vi "OAT_Display_Freq-RPM Map.vi"(9 "Gabor Template":dbl[](array[numeric]) format="%.2f", 10 "sampling frequency (Hz)":dbl, 11 "Gabor RefNum":T1) -> (1 "Diagram":picture, 2 "Freq-RPM Map":u8[][](graph), 3 "Gabor RefNum Out":T1, 4 "Diagram":bool, 5 "Order":dbl=1.0 format="%.1f")   [LabVIEW 2017]
doc: "This VI is a sub-window of Order Analyzer. It displays RPM-Order map in intensity graph and waterfall plot."
uses:
  <vilib>/addons/Sound and Vibration/Order Analysis/Ref Gabor Order Tracking/GT RefNum.ctl
  <vilib>/addons/Sound and Vibration/Order Analysis/Ref Gabor Order Tracking/Get Freq-RPM Spectral Map (DBL).vi
  <vilib>/addons/Sound and Vibration/Order Analysis/Ref Gabor Order Tracking/Get Freq-RPM Spectral Map (U8).vi
  <vilib>/addons/Sound and Vibration/Order Analysis/Gabor Order Tracking/SoundVib_Gabor.lvlib
panel:
  in  "help mask":cluster{"OK Button":bool}
  in  "Help":bool
  out "Cursor Mask":cluster{dbl, dbl}[](graph)
  in  "stop":bool
  in  "[user-specified font]":T2={"Font Name:"="MS Sans Serif", "Size"=13, "Strikeout?"=FALSE, "Italic?"=FALSE, "Underline?"=FALSE, "Outline?"=FALSE, "Shadow?"=FALSE, "Bold?"=FALSE}
  in  "Order Info":T3={"Lowest order"=1.0, "# of Orders"=20.0, "Resolution"=0.1} {"Resolution" format="%.2f"; "# of Orders" format="%.1f"; "Lowest order" format="%.1f"}
  in  "dB ON":bool=TRUE
  in  "Waterfall ColorMap":i32(ring)=2 items=["cwNone", "cwShaded", "cwColorSpectrum", "cwGrayScale"]
  out "status":string
  in  "Diagram\n\nIntensity":bool
  # "1. Zoom Intensity Graph by setting ranges of axis.\n\n2. Switch to Diagram to display Campbell diagram.\n\n3. Move the cursor to find out which order the engergy consentrats on.\n\nClick on this screen to continue"
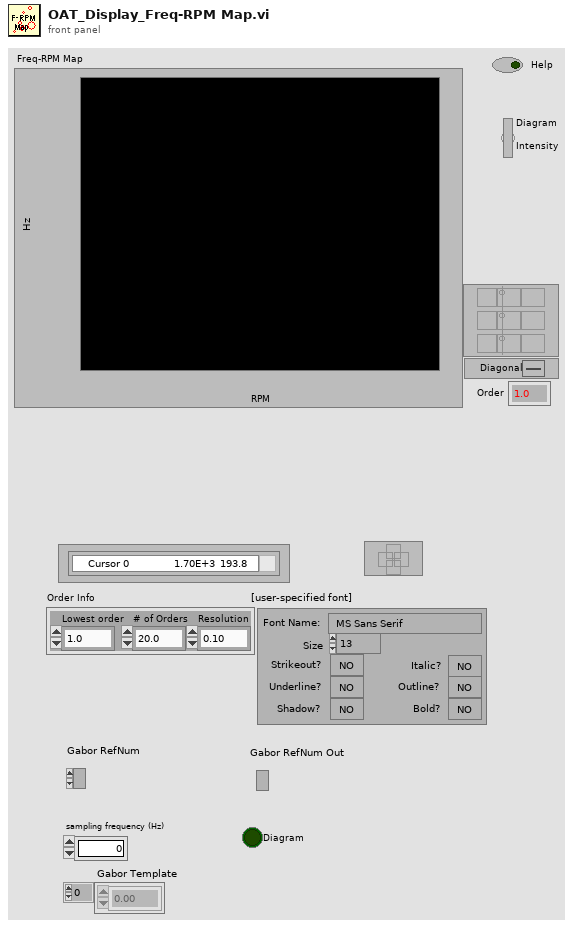
[diagram p1: front panel]
types:
  T1 = typedef "SoundVib_Gabor.lvlib/GT RefNum.ctl" = refnum<k1>
  T2 = cluster{"Font Name:":string, "Size":i16, "Strikeout?":bool, "Italic?":bool, "Underline?":bool, "Outline?":bool, "Shadow?":bool, "Bold?":bool}
  T3 = cluster{"Lowest order":dbl, "# of Orders":dbl, "Resolution":dbl}
  T4 = enum16{"User-specified Font", "Application Font", "System Font", "Dialog Font"}
  T5 = cluster{"x minimum":dbl, "x maximum":dbl, "x log?":bool, "x precision":u8, "x format":enum8{"Decimal", "Scientific", "Engineering", "Binary", "Octal", "Hex"}, "y minimum":dbl, "y maximum":dbl, "y log?":bool, "y precision":u8, "y format":enum8{"Decimal", "Scientific", "Engineering", "Binary", "Octal", "Hex"}}
  T6 = cluster{"Gabor RefNum":T1, "dB ON":bool, "Order Info":cluster{"Lowest order":dbl, "# of Orders":dbl, "Resolution":dbl}}
  T7 = cluster{"Diagram\n\nIntensity":bool, "Waterfall ColorMap":i32}
  T8 = typedef "LVBoundsTypeDef.ctl" = cluster{"Width":u32, "Height":u32}
  T9 = cluster{"x [EU]":dbl, "y [EU]":dbl, "radius [pixel]":dbl}[]
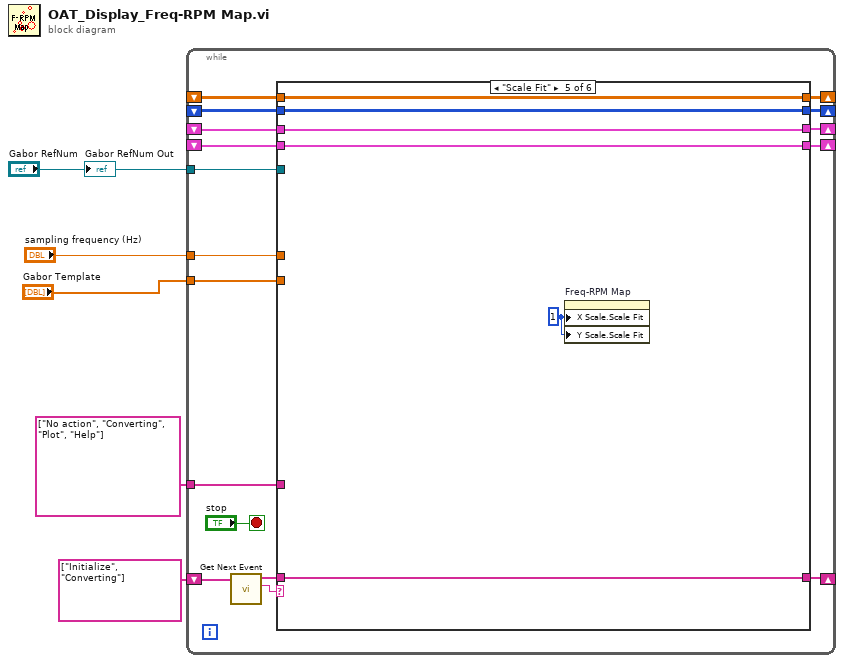
[diagram p0: block diagram]
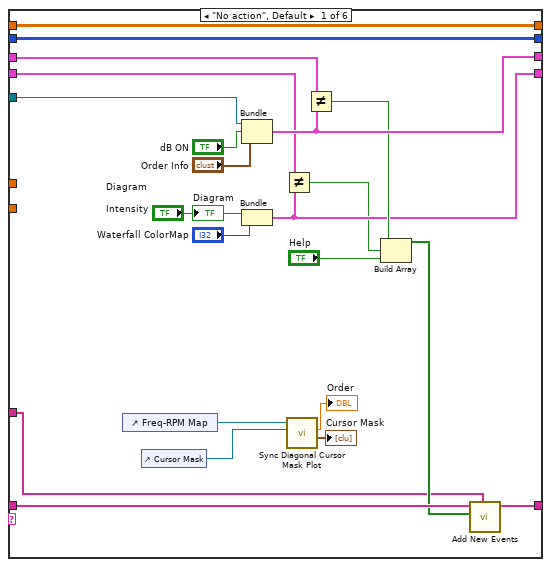
[diagram p2: hidden frame]
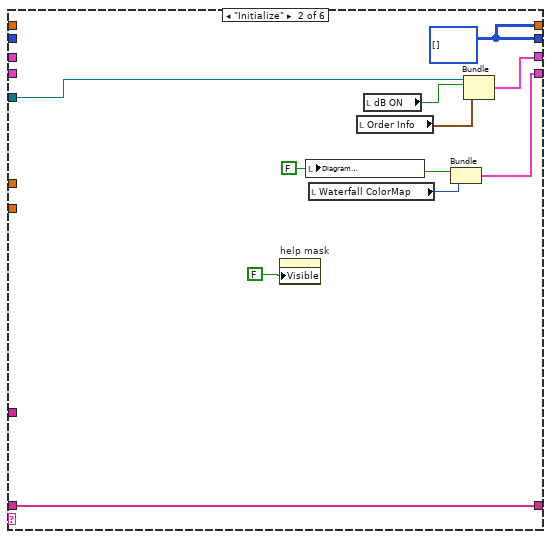
[diagram p3: hidden frame]
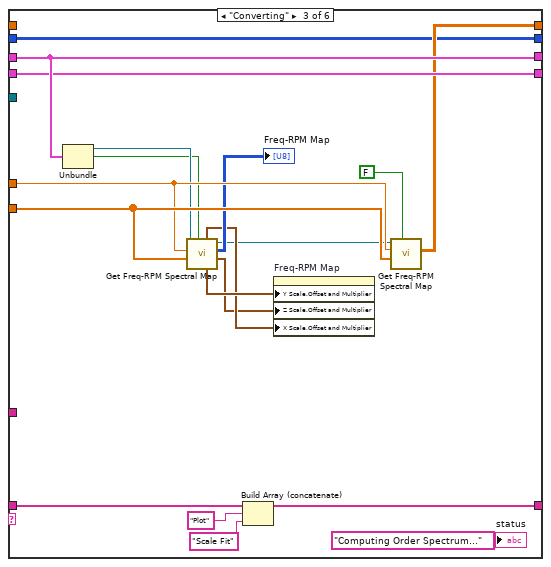
[diagram p4: hidden frame]
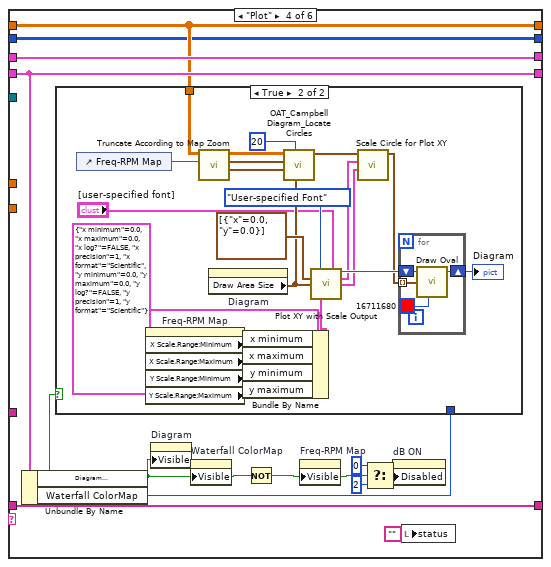
[diagram p5: hidden frame]
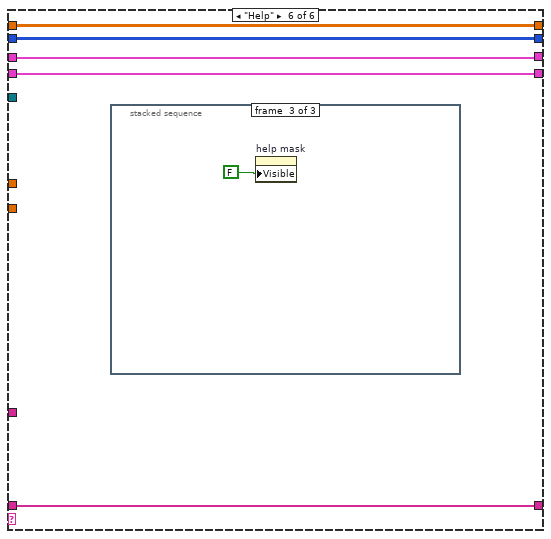
[diagram p7: hidden frame]
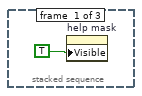
[diagram p8: hidden frame]
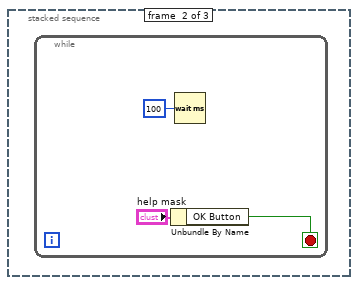
[diagram p9: hidden frame]
diagram:
  n1 = while {
    tunnel: "Gabor Template" -> [w7]
    tunnel: "sampling frequency (Hz)" -> [w8]
    tunnel: "Gabor RefNum" -> [w9]
    shift-left: _ -> [w10]
    shift-right: [w11] -> _
    tunnel: string[] ["No action", "Converting", "Plot", "Help"] ("Event Queue Out") -> [w12]
    shift-left: _ -> [w14]
    shift-right: [w13] -> _
    shift-left: _ -> [w15]
    shift-right: [w16] -> _
    shift-left: _ -> [w17]
    shift-right: [w18] -> _
    shift-left: string[] ["Initialize", "Converting"] ("Event Queue Out") -> [w19]
    shift-right: [w22] -> _
    stop <- "stop" stop-if-true
    n2 = call <vilib>:"Get Next Event.vi"("Event Queue In"=w19) -> ("Next Event"=w20:string, "Event Queue Out"=w21:string[])  [unwired: 5 in]
    n3 = case shown="\"Scale Fit\"" w20 {
      tunnel: [w44 w47 w65 w74 w116 w121] -> w18
      tunnel: w17 -> [w44 _ w65 w74 w116 w121]
      tunnel: [w43 w54 w71 w84 w113 w118] -> w22
      tunnel: w21 -> [w42 w54 w73 w84 w113 w118]
      tunnel: [w40 w52 w70 w80 w115 w120] -> w16
      tunnel: w15 -> [w39 _ w70 w80 w115 w120]
      tunnel: w14 -> [w35 _ w68 w85 w114 w119]
      tunnel: [w34 w49 w68 w85 w114 w119] -> w13
      tunnel: w12 -> [w31 _ _ _ _ _]
      tunnel: [w25 w47 w66 w78 w117 w122] -> w11
      tunnel: w10 -> [w25 _ _ w78 w117 w122]
      tunnel: w9 -> [w23 w45 _ _ _ _]
      tunnel: w8 -> [_ _ w64 _ _ _]
      tunnel: w7 -> [_ _ w67 _ _ _]
      frame "No action", Default {
        n4 = control-ref of="Freq-RPM Map"() -> (w29:refnum<vi>)
        n5 = control-ref of="Cursor Mask"() -> (w28:refnum<vi>)
        n6 = Bundle("Gabor RefNum"=w23, "dB ON"="dB ON", "Order Info"="Order Info") -> (w40:T6)  [unwired: 1 in]
        n7 = Bundle("Diagram\n\nIntensity"="Diagram\n\nIntensity", "Waterfall ColorMap"="Waterfall ColorMap") -> (w34:T7)  [unwired: 1 in]
        n8 = Not Equal?(x=w35, y=w34) -> (x != y?=w32:bool)
        n9 = call <vilib>:"Sync Diagonal Cursor Mask Plot.vi"("Cursor Mask"=w28, "Freq-RPM Map"=w29) -> ("diagonal line"=→"Cursor Mask":cluster{dbl, dbl}[], "order number"=→"Order":dbl)  [unwired: 7 in, 1 out]
        n10 = Not Equal?(x=w39, y=w40) -> (x != y?=w38:bool)
        n11 = Build Array(w38, w32, "Help") -> (w33:bool[])
        n12 = call <vilib>:"Add New Events.vi"("Event Names"=w31, "New Events"=w33, "Event Queue In"=w42) -> ("Event Queue Out"=w43:string[])  [unwired: 8 in]
        "Diagram" <- "Diagram\n\nIntensity"
      }
      frame "Initialize" {
        w50 = FALSE ("Diagram\n\nIntensity")
        w47 = u8[][] [] ("Graph Data [U8]")
        n13 = property on="help mask" class="Clust"("Visible"=FALSE) -> ()  [unwired: 2 in, 2 out]
        n14 = local write "Diagram\n\nIntensity"(w50) -> ()
        n15 = local read "Waterfall ColorMap"() -> (w51:i32)
        n16 = local read "Order Info"() -> (w48:T3)
        n17 = local read "dB ON"() -> (w53:bool)
        n18 = Bundle("Diagram\n\nIntensity"=w50, "Waterfall ColorMap"=w51) -> (w49:T7)  [unwired: 1 in]
        n19 = Bundle("Gabor RefNum"=w45, "dB ON"=w53, "Order Info"=w48) -> (w52:T6)  [unwired: 1 in]
      }
      frame "Converting" {
        n20 = Unbundle(w70) -> ("Gabor RefNum"=w60:T1, "dB ON"=w57:bool)  [unwired: 1 out]
        n21 = call-poly <vilib>:"Get Freq-RPM Spectral Map.vi"("dB On (T)"=w57, "Gabor template"=w67, "sampling frequency [Hz]"=w64, "RefNum in"=w60) -> ("quantization info"=w56:cluster{"offset":dbl, "multiplier":dbl}, "spectral map"=→"Freq-RPM Map":u8[][], "RefNum out"=w59:T1, "frequency scale"=w62:cluster{"offset":dbl, "multiplier":dbl}, "rpm scale"=w61:cluster{"offset":dbl, "multiplier":dbl})  [unwired: 2 in, 1 out]
        n22 = Build Array (concatenate)(w73, "Plot" ("status"), "Scale Fit" ("status")) -> (w71:string[])
        n23 = property on="Freq-RPM Map" class="IntGraph (strict)"("Y Scale.Offset and Multiplier"=w62, "Z Scale.Offset and Multiplier"=w56, "X Scale.Offset and Multiplier"=w61) -> ()  [unwired: 2 in, 2 out]
        n24 = call-poly <vilib>:"Get Freq-RPM Spectral Map.vi"("dB On (T)"=FALSE, "Gabor template"=w67, "sampling frequency [Hz]"=w64, "RefNum in"=w59) -> ("spectral map"=w66:dbl[][])  [unwired: 2 in, 5 out]
        "status" <- "Computing Order Spectrum..."
      }
      frame "Plot" {
        n25 = Unbundle By Name(w85) -> ("Diagram\n\nIntensity"=w81:bool, "Waterfall ColorMap"=w82:i32)
        n26 = case shown="True" w81 {
          tunnel: w78 -> [_ w89]
          tunnel: w82 -> [_ _]
          frame False {
          }
          frame True {
            n27 = control-ref of="Freq-RPM Map"() -> (w90:refnum<vi>)
            n28 = property on="Freq-RPM Map" class="IntGraph (strict)"() -> ("X Scale.Range:Minimum"=w107:dbl, "X Scale.Range:Maximum"=w106:dbl, "Y Scale.Range:Minimum"=w105:dbl, "Y Scale.Range:Maximum"=w104:dbl)  [unwired: 2 in, 2 out]
            n29 = call <vilib>:"Truncate According to Map Zoom.vi"("Map reference"=w90, "data"=w89) -> ("Y Scale.Offset and Multiplier"=w86:cluster{"Offset":dbl, "Multiplier":dbl}, "X Scale.Offset and Multiplier"=w87:cluster{"Offset":dbl, "Multiplier":dbl}, "data out"=w88:dbl[][])  [unwired: 7 in]
            n30 = property on="Diagram" class="Pict"() -> ("Draw Area Size"=w96:T8)  [unwired: 2 in, 2 out]
            n31 = Bundle By Name(cluster=T5 {"x minimum"=0.0, "x maximum"=0.0, "x log?"=FALSE, "x precision"=1, "x format"=enum."Scientific", "y minimum"=0.0, "y maximum"=0.0, "y log?"=FALSE, "y precision"=1, "y format"=enum."Scientific"} ("cartesian axis attributes"), "x minimum"=w107, "x maximum"=w106, "y minimum"=w105, "y maximum"=w104) -> (w103:T5)
            n32 = call <vilib>:"OAT_Campbell Diagram_Locate Circles.vi"("picture size (w,h)"=w96, "number of x steps"=20, "y scale"=w86, "x scale"=w87, "map"=w88) -> ("circles"=w95:T9)  [unwired: 6 in]
            n33 = call <vilib>:"Plot XY with Scale Output.vi"("desired font(Application)"=T4."User-specified Font", "[user-specified font]"="[user-specified font]", "data"=cluster{"x":dbl, "y":dbl}[] [{"x"=0.0, "y"=0.0}], "dimensions (w,h)"=w96, "cartesian axis attributes"=w103) -> ("new picture"=w101:picture, "x scale factors"=w99:cluster{"a":dbl, "b":dbl, "log?":bool}, "y scale factors"=w98:cluster{"a":dbl, "b":dbl, "log?":bool})  [unwired: 8 in]
            n34 = call <vilib>:"Scale Circle for Plot XY.vi"("y scale factors"=w98, "x scale factors"=w99, "circles"=w95) -> ("rectangles"=w97:cluster{i16, i16, i16, i16}[])  [unwired: 8 in]
            n35 = for {
              shift-right: [w110] -> w100
              shift-left: w101 -> [w111]
              tunnel: w97 -> [w109] mode=indexing
              n36 = call <vilib>:"Draw Oval.vi"("picture"=w111, "rect"=w109, "color(black)"=u32 16711680) -> ("new picture"=w110:picture)  [unwired: 6 in]
            }
            "Diagram" <- w100
          }
        }
        n37 = property on="Diagram" class="Pict"("Visible"=w81) -> ()  [unwired: 2 in, 2 out]
        n38 = property on="Waterfall ColorMap" class="Ring (strict)"("Visible"=w81) -> ()  [unwired: 2 in, 2 out]
        n39 = Not(x=w81) -> (.not. x?=w79:bool)
        n40 = property on="Freq-RPM Map" class="IntGraph (strict)"("Visible"=w79) -> ()  [unwired: 2 in, 2 out]
        n41 = Select(t=0, s=w79, f=2) -> (s? t:f=w77:i32)
        n42 = property on="dB ON" class="Bool (strict)"("Disabled"=w77) -> ()  [unwired: 2 in, 2 out]
        n43 = local write "status"("") -> ()
      }
      frame "Scale Fit" {
        w112 = u8 1 ("X Scale.Scale Fit")
        n44 = property on="Freq-RPM Map" class="IntGraph (strict)"("X Scale.Scale Fit"=w112, "Y Scale.Scale Fit"=w112) -> ()  [unwired: 2 in, 2 out]
      }
      frame "Help" {
        n45 = stacked-sequence {
          frame #0 {
            n46 = property on="help mask" class="Clust"("Visible"=TRUE) -> ()  [unwired: 2 in, 2 out]
          }
          frame #1 {
            n47 = while {
              stop <- w125 stop-if-true
              n48 = Unbundle By Name("help mask") -> ("OK Button"=w125:bool)
              n49 = Wait (ms)(milliseconds to wait=u32 100) -> ()  [unwired: 1 out]
            }
          }
          frame #2 {
            n50 = property on="help mask" class="Clust"("Visible"=FALSE) -> ()  [unwired: 2 in, 2 out]
          }
        }
      }
    }
  }
  "Gabor RefNum Out" <- "Gabor RefNum"
